vi "SetParam.vi"(8 "error in (no error)":errorcluster caption="entrée d'erreur (pas d'erreur)", 10 "OneHotEncoder":T1={"drop"="None", "sparse"=TRUE, "dtype"="float", "handle_unknown"="error"}, 11 "OneHotEncoder.lvclass":refnum<class "OneHotEncoder.lvclass">) -> (0 "error out":errorcluster caption="sortie d'erreur", 3 "OneHotEncoder.lvclass":refnum<class "OneHotEncoder.lvclass">)   [LabVIEW 2020, in "OneHotEncoder.lvclass"]
doc: "Set Parameters"
uses:
  OneHotEncoder.lvclass
  OneHotEncoder.lvclass/OneHotEncoder.ctl
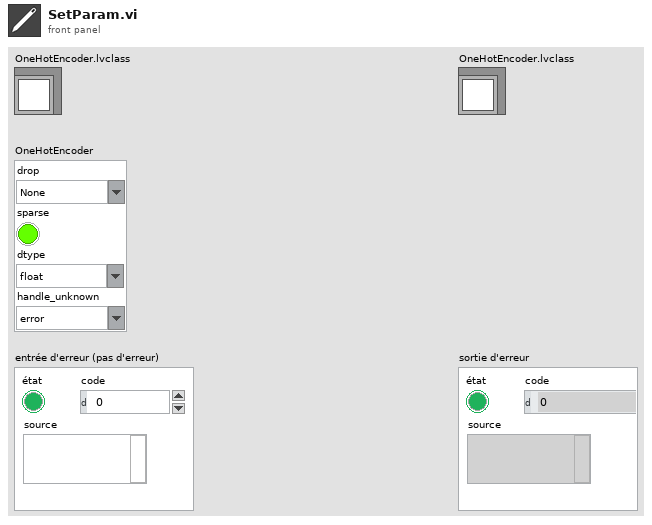
[diagram p1: front panel]
types:
  T1 = cluster{"drop":string, "sparse":bool, "dtype":string, "handle_unknown":string}
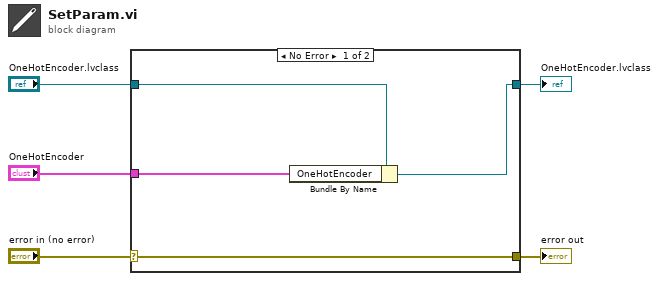
[diagram p0: block diagram]
diagram:
  n1 = case shown="No Error" "error in (no error)" {
    selector: "error in (no error)" -> [w9 w10]
    tunnel: [w9 w10] -> w4
    tunnel: [w7 w11] -> w2
    tunnel: "OneHotEncoder.lvclass" -> [w8 w11]
    tunnel: "OneHotEncoder" -> [w6 _]
    frame No Error {
      n2 = Bundle By Name(cluster=w8, "OneHotEncoder"=w6) -> (w7:refnum<class "OneHotEncoder.lvclass">)
    }
    frame Error {
    }
  }
  "error out" <- w4
  "OneHotEncoder.lvclass" <- w2
